vi "CloseVIReference.vi"(3 "VI Refnum":refnum<vi>) -> ()   [LabVIEW 2012]
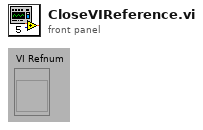
[diagram p1: front panel]
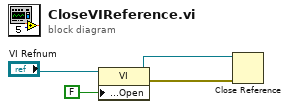
[diagram p0: block diagram]
diagram:
  n1 = property class="VI"(reference="VI Refnum", "Front Panel Window:Open"=FALSE) -> (reference out=w2:refnum<vi>, error out=w1:errorcluster)  [unwired: 1 in]
  n2 = Close Reference(reference=w2, error in (no error)=w1) -> ()  [unwired: 1 out]
